vi "Error Handler - Message Handling Loop_.vi"(8 "error in (no error)":errorcluster) -> (0 "error dup":errorcluster, 5 "channel":T1)   [LabVIEW 2023]
uses:
  Message Queue.lvlib
  Message Cluster.ctl
  <extravilib>/ChannelInstances/Messenger-t'Message Queue.lvlib-Message Cluster.ctl'/))Channel.ctl
  <extravilib>/ChannelInstances/Messenger-t'Message Queue.lvlib-Message Cluster.ctl'.lvlib
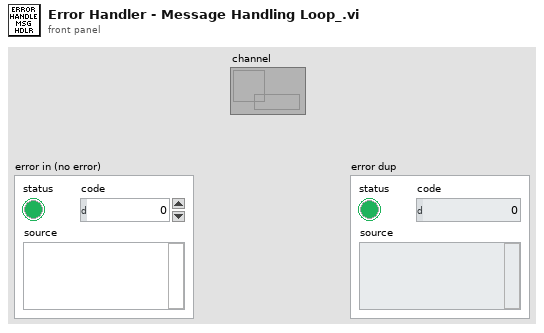
[diagram p1: front panel]
types:
  T1 = typedef "Messenger-t'Message Queue.lvlib-Message Cluster.ctl'.lvlib/))Channel.ctl" = refnum<queue>
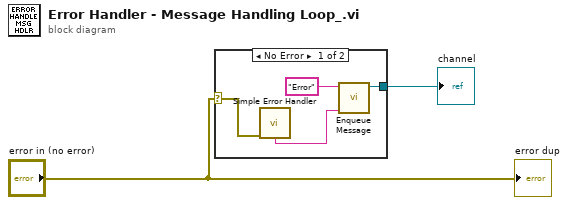
[diagram p0: block diagram]
diagram:
  n1 = case shown="No Error" "error in (no error)" {
    selector: "error in (no error)" -> [w5 _]
    tunnel: [w3 _] -> w1
    frame No Error {
      n2 = call <vilib>:"Simple Error Handler.vi"("error in (no error)"=w5) -> ("message"=w4:string)  [unwired: 4 in, 4 out]
      n3 = call "Enqueue Message.vi"("Message Data"=w4, "Message"="Error") -> ("channel"=w3:T1)  [unwired: 9 in]
    }
    frame Error {
    }
  }
  "channel" <- w1
  "error dup" <- "error in (no error)"
